vi "結束畫面.vi"(2 "Numeric":dbl) -> (0 "結束遊戲 2":bool, 1 "再玩一次 2":bool)   [LabVIEW 2014]
panel:
  in  "結束遊戲":bool
  in  "再玩一次":bool
  # "本次遊戲獲得分數為："
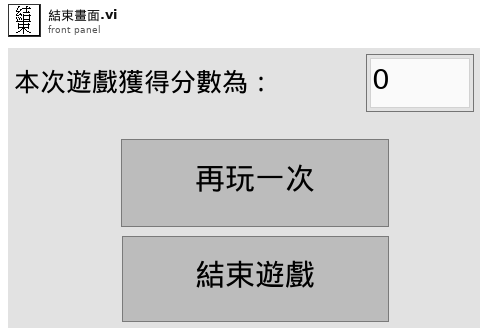
[diagram p1: front panel]
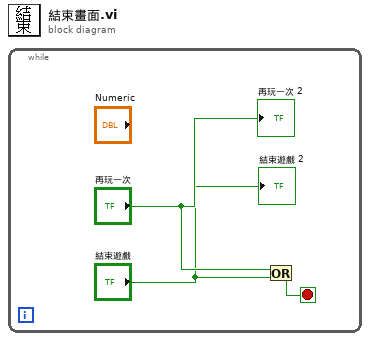
[diagram p0: block diagram]
diagram:
  n1 = while {
    stop <- w1 stop-if-true
    n2 = Or(x="再玩一次", y="結束遊戲") -> (x .or. y?=w1:bool)
    "再玩一次 2" <- "再玩一次"
    "結束遊戲 2" <- "結束遊戲"
  }
